vi "Client.vi"() -> ()   [LabVIEW 2020]
uses:
  Server/_support/Module/typedef/tcp-msg type.ctl
  <vilib>/event_ctls.llb/eventvkey.ctl
  a1c83761-5f2f-4742-9fa6-a9430ba65f56.vi
  <userlib>/_NEVSTOP/Communicable State Machine(CSM)/_Support/Common/Trim Single line Text.vi
  <userlib>/_NEVSTOP/Communicable State Machine(CSM)/AdvanceAPI/CSM - Keywords.vi
  <userlib>/_NEVSTOP/Communicable State Machine(CSM)/Communicable State Machine.lvlib
  <userlib>/_NEVSTOP/Communicable State Machine(CSM)/addons/API-String-Arugments-Support/API String Arguments Support.lvlib
  <userlib>/_NEVSTOP/Communicable State Machine(CSM)/addons/INI-Static-Variable-Support/INI-Static-Variable-Support.lvlib
  Server/_support/Module/CSM-TCP-Router.lvlib
panel:
  out "exit":bool
  out "Console":string
  in  "Command":string caption="$"
  out "To Who":string
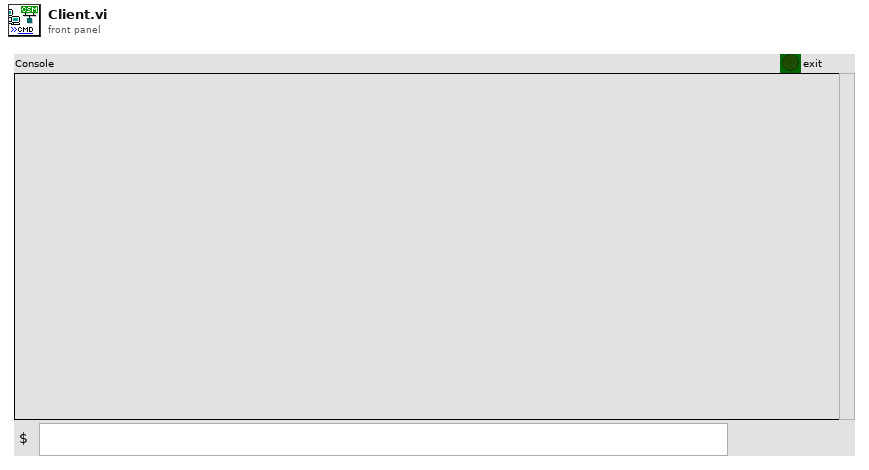
[diagram p1: front panel]
types:
  T1 = typedef "CSM-TCP-Router.lvlib/tcp-msg type.ctl" = enum8{"info", "error", "cmd", "resp", "async-resp", "status", "interrupt"}
  T2 = typedef "eventvkey.ctl" = enum16{"ASCII", "Enter", "Return", "Shift", "Ctrl", "Alt", "Cmd", "Opt", "Caps", "NumLock", "Clear", "Break", "Up", "Down", "Left", "Right", "Insert", "Delete", "Home", "End", "PageUp", "PageDown", "Escape", "Help", "Pause", "ScrollLock", "F1", "F2", "F3", "F4", "F5", "F6", "F7", "F8", "F9", "F10", "F11", "F12", "F13", "F14", "F15", "F16", "F17", "F18", "F19", "F20", "F21", "F22", "F23", "F24", "Play", "VolumeUp", "VolumeDown", "Mute", "Two Byte Char"}
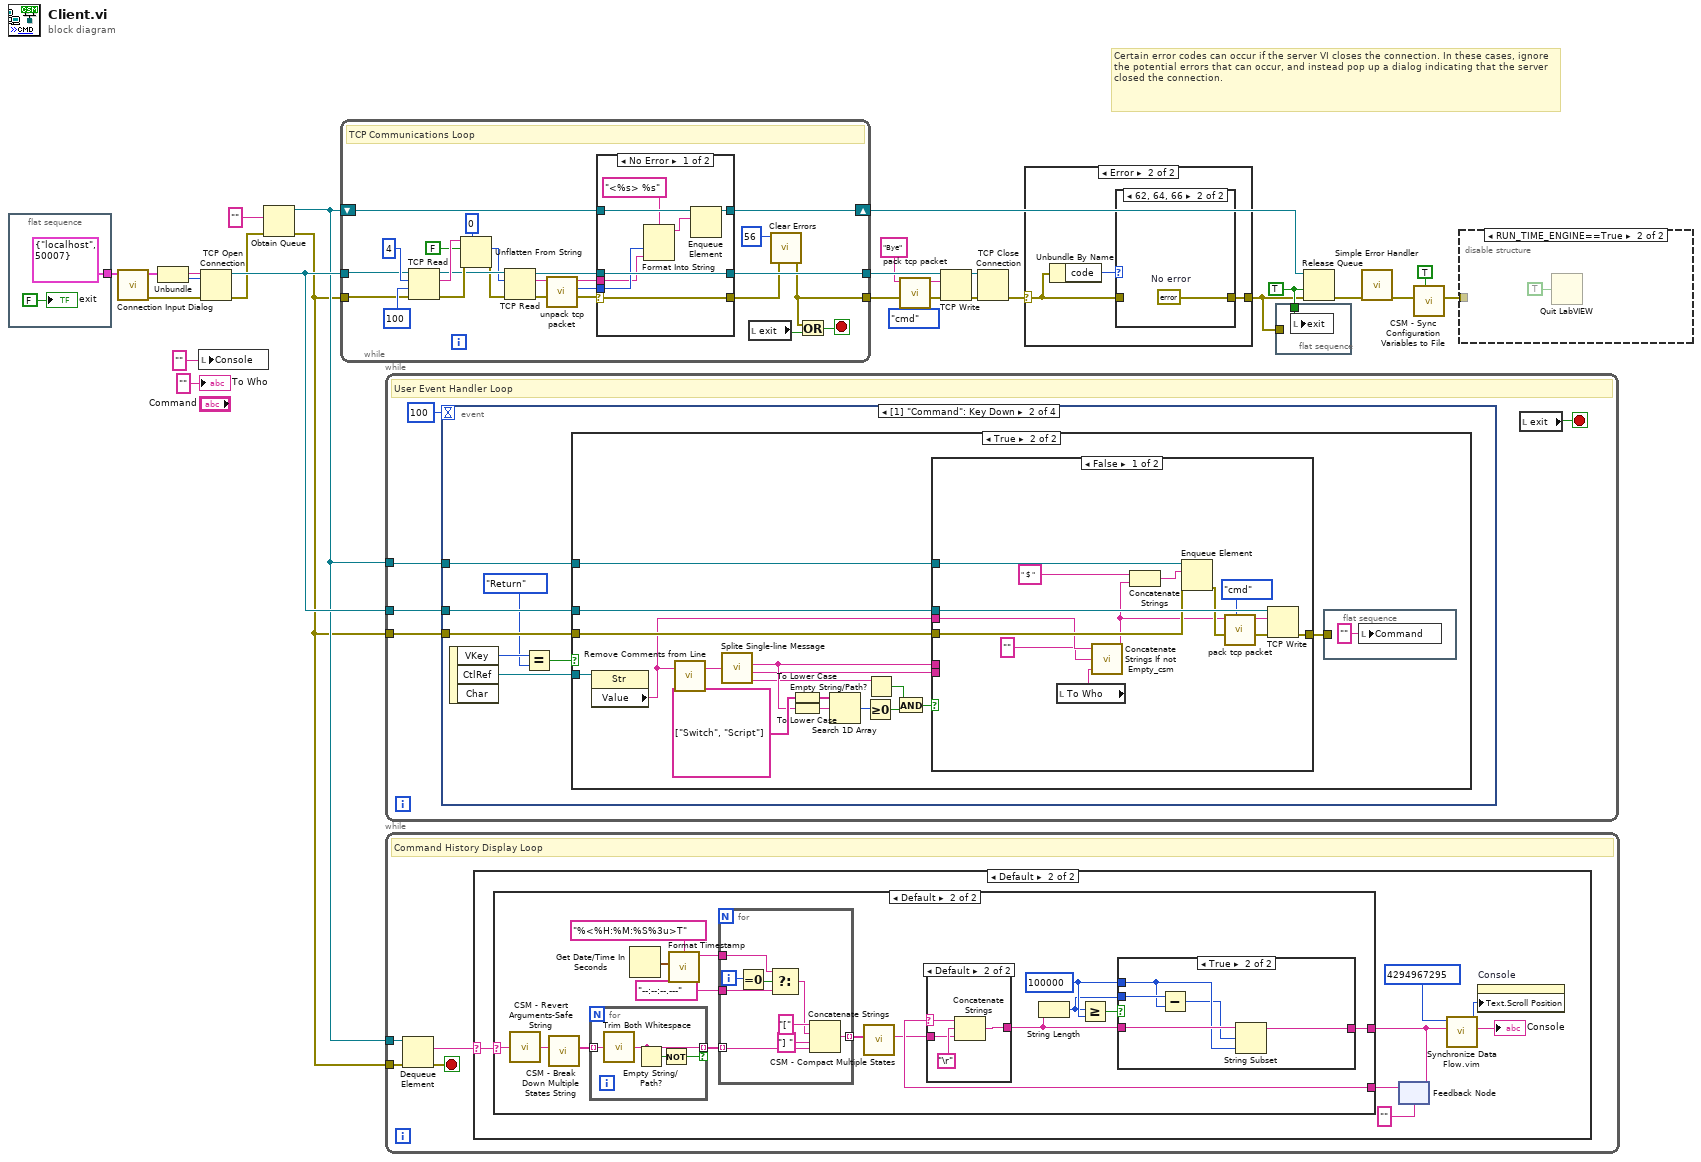
[diagram p0: block diagram]
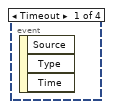
[diagram p7: hidden frame]
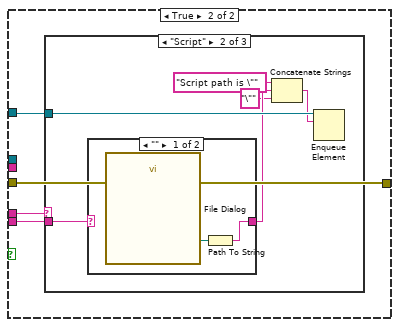
[diagram p9: hidden frame]
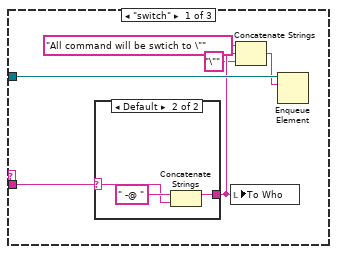
[diagram p10: hidden frame]
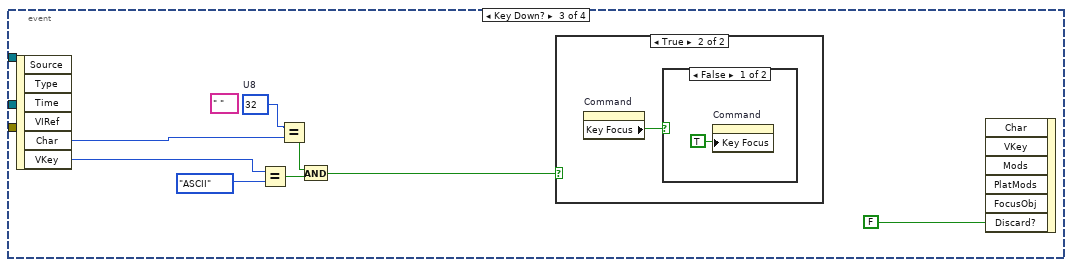
[diagram p14: hidden frame]
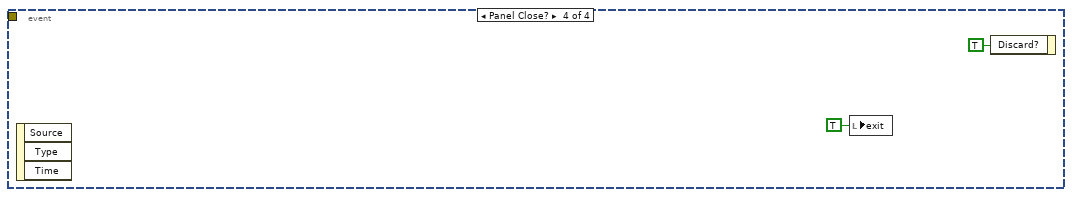
[diagram p17: hidden frame]
diagram:
  w6 = TRUE ("force destroy? (F)")
  # "Certain error codes can occur if the server VI closes the connection. In these cases, ignore the potential errors that can occur, and instead pop up a dialog indicating that the server closed the connection."
  n1 = flat-sequence {
    tunnel: [cluster{"IP Address":string, "Port":u16} {"IP Address"="localhost", "Port"=50007} ("Connection Info")] -> w16
    frame #0 {
      "exit" <- FALSE ("exit")
    }
  }
  n2 = call "Connection Input Dialog.vi"("Connection Info"=w16) -> ("Error out"=w15:errorcluster, "Connection Info output"=w14:cluster{"IP Address":string, "Port":u16})  [unwired: 9 in]
  n3 = Unbundle(w14) -> ("IP Address"=w13:string, "Port"=w12:u16)
  n4 = local write "Console"("" ("data out")) -> ()
  n5 = TCP Open Connection(address=w13, remote port or service name=w12, error in (no error)=w15) -> (connection ID=w21:refnum<k5>, error out=w9:errorcluster)  [unwired: 2 in]
  n6 = Obtain Queue(element data type="" ("name (unnamed)"), error in (no error)=w9) -> (queue out=w19:refnum<queue>, error out=w8:errorcluster)  [unwired: 3 in, 1 out]
  n7 = while {
    tunnel: w8 -> [w34]
    tunnel: w21 -> [w35]
    tunnel: [w53] -> w26
    tunnel: [w47] -> w24
    shift-right: [w49] -> w7
    shift-left: w19 -> [w50]
    stop <- w48 stop-if-true
    # "TCP Communications Loop"
    n8 = TCP Read(connection ID=w35, bytes to read=4, error in (no error)=w34, 9:100 ("timeout ms (1000)")) -> (connection ID out=w43:refnum<k5>, data out=w44:string, error out=w45:errorcluster)  [unwired: 1 in]
    n9 = Unflatten From String(type=0, binary string=w44, data includes array or string size? (T)=FALSE, error in (no error)=w45) -> (value=w41:i32, error out=w40:errorcluster)  [unwired: 2 out]
    n10 = TCP Read(connection ID=w43, bytes to read=w41, error in (no error)=w40) -> (connection ID out=w32:refnum<k5>, data out=w42:string, error out=w33:errorcluster)  [unwired: 2 in]
    n11 = call "unpack tcp packet.vi"("TCP Pack"=w42) -> ("tcp-message-type"=w30:T1, "String"=w31:string)  [unwired: 9 in]
    n12 = case shown="No Error" w33 {
      selector: w33 -> [w60 w64]
      tunnel: w32 -> [w61 w63]
      tunnel: [w61 w63] -> w53
      tunnel: [w60 w64] -> w52
      tunnel: w31 -> [w56 _]
      tunnel: w50 -> [w59 w62]
      tunnel: [w58 w62] -> w49
      tunnel: w30 -> [w57 _]
      frame No Error {
        n13 = Format Into String(format string="<%s> %s", w57, w56) -> (resulting string=w55:string)  [unwired: 2 in, 1 out]
        n14 = Enqueue Element(queue=w59, element=w55) -> (queue out=w58:refnum<queue>)  [unwired: 2 in, 2 out]
      }
      frame Error {
      }
    }
    n15 = local read "exit"() -> (w46:bool)
    n16 = call <vilib>:"Clear Errors.vi"("error in (no error)"=w52, "specific error code to clear (0: all)"=56) -> ("error out"=w47:errorcluster)  [unwired: 4 in, 1 out]
    n17 = Or(x=w47, y=w46) -> (x .or. y?=w48:bool)
  }
  n18 = while {
    tunnel: w21 -> [w69]
    tunnel: w8 -> [w68]
    tunnel: w19 -> [w66]
    stop <- w65 stop-if-true
    # "User Event Handler Loop"
    n19 = event shown="[1] \"Command\": Key Down" {
      selector: _ -> [_ _ _ _]
      dyn-events: _ -> [_ _ _ _]
      timeout: 100 -> [_ _ _ _]
      tunnel: w69 -> [_ w76 _ _]
      tunnel: w68 -> [_ w74 _ _]
      tunnel: w66 -> [_ w75 _ _]
      event Timeout {
        n20 = event-data() -> ()  [unwired: 1 in, 3 out]
      }
      event "Command": Key Down {
        n21 = event-data() -> ("VKey"=w72:T2, "CtlRef"=w73:refnum<vi>)  [unwired: 1 in, 1 out]
        n22 = Equal?(x=w72, y=eventvkey."Return") -> (x = y?=w70:bool)
        n23 = case shown="True" w70 {
          tunnel: w76 -> [_ w93]
          tunnel: w75 -> [_ w92]
          tunnel: w74 -> [_ w91]
          tunnel: w73 -> [_ w90]
          frame False {
          }
          frame True {
            n24 = property class="Str"(reference=w90) -> ("Value"=w87:string)  [unwired: 1 in, 2 out]
            n25 = call <userlib>:"Remove Comments from Line.vi"("single-line text"=w87) -> ("single-line text without comments"=w88:string)  [unwired: 2 in]
            n26 = call <userlib>:"Splite Single-line Message.vi"("single-line text"=w88) -> ("state"=w85:string, "args"=w77:string, "source/target"=w78:string)  [unwired: 6 in, 1 out]
            n27 = To Lower Case(string=string[] ["Switch", "Script"] ("hostname")) -> (all lower case string=w80:string[])
            n28 = To Lower Case(string=w85) -> (all lower case string=w79:string)
            n29 = Search 1D Array(1D array=w80, element=w79) -> (index of element=w84:i32)  [unwired: 1 in]
            n30 = Greater Or Equal To 0?(x=w84) -> (x >= 0?=w83:bool)
            n31 = Empty String/Path?(string/path=w78) -> (empty?=w82:bool)
            n32 = And(x=w82, y=w83) -> (x .and. y?=w81:bool)
            n33 = case shown="False" w81 {
              tunnel: w93 -> [w106 _]
              tunnel: w92 -> [w105 w109]
              tunnel: w91 -> [w101 w110]
              tunnel: [w100 w110] -> w89
              tunnel: w87 -> [w99 _]
              tunnel: w85 -> [_ w107]
              tunnel: w77 -> [_ w108]
              frame False {
                n34 = local read "To Who"() -> (w96:string)
                n35 = call <userlib>:"Concatenate Strings If not Empty_csm.vi"("String"=w96, "seperator(:)"="", "prefix"=w99) -> ("result"=w98:string)  [unwired: 2 in]
                n36 = Concatenate Strings(" $ " ("string"), w98) -> (w103:string)
                n37 = Enqueue Element(queue=w105, element=w103, error in (no error)=w101) -> (error out=w102:errorcluster)  [unwired: 1 in, 2 out]
                n38 = call "pack tcp packet.vi"("tcp-message-type"=tcp-msg_type."cmd", "String"=w98) -> ("TCP Pack"=w95:string)  [unwired: 9 in]
                n39 = TCP Write(connection ID=w106, data in=w95, error in (no error)=w102) -> (error out=w100:errorcluster)  [unwired: 1 in, 2 out]
              }
              frame True {
                n40 = case shown="\"Script\"" w107 {
                  tunnel: w109 -> [w115 w124 _]
                  tunnel: w108 -> [w116 w125 _]
                  frame "switch" {
                    n41 = case shown="Default" w116 {
                      selector: w116 -> [_ w117]
                      tunnel: [_ w118] -> w114
                      frame "" {
                      }
                      frame Default {
                        n42 = Concatenate Strings(" -@ " ("To Who"), w117) -> (w118:string)
                      }
                    }
                    n43 = local write "To Who"(w114) -> ()
                    n44 = Concatenate Strings("All command will be swtich to \"" ("string"), w114, "\"" ("string")) -> (w113:string)
                    n45 = Enqueue Element(queue=w115, element=w113) -> ()  [unwired: 2 in, 3 out]
                  }
                  frame "Script" {
                    n46 = case shown="\"\"" w125 {
                      selector: w125 -> [_ w128]
                      tunnel: [w126 w128] -> w123
                      frame "" {
                        n47 = call "File Dialog"() -> ("selected path"=w127:path)  [unwired: 12 in, 3 out]
                        n48 = Path To String(path=w127) -> (string=w126:string)
                      }
                      frame Default {
                      }
                    }
                    n49 = Concatenate Strings("Script path is \"" ("string"), w123, "\"" ("string")) -> (w122:string)
                    n50 = Enqueue Element(queue=w124, element=w122) -> ()  [unwired: 2 in, 3 out]
                  }
                  frame Default {
                  }
                }
              }
            }
            n51 = flat-sequence {
              tunnel: w89 -> [_]
              frame #0 {
                n52 = local write "Command"("" ("Command")) -> ()
              }
            }
          }
        }
      }
      event Key Down? {
        (unwired) " "
        w132 = u8 32  # U8
        n53 = event-data() -> ("Char"=w133:i16, "VKey"=w135:T2)  [unwired: 1 in, 4 out]
        n54 = Equal?(x=w135, y=eventvkey."ASCII" ("VKey")) -> (x = y?=w134:bool)
        n55 = Equal?(x=w132, y=w133) -> (x = y?=w131:bool)
        n56 = And(x=w131, y=w134) -> (x .and. y?=w130:bool)
        n57 = case shown="True" w130 {
          frame False {
          }
          frame True {
            n58 = property on="Command" class="Str"() -> ("Key Focus"=w138:bool)  [unwired: 2 in, 2 out]
            n59 = case shown="False" w138 {
              frame False {
                n60 = property on="Command" class="Str"("Key Focus"=TRUE) -> ()  [unwired: 2 in, 2 out]
              }
              frame True {
              }
            }
          }
        }
        n61 = event-data("Discard?"=FALSE) -> ()  [unwired: 6 in, 1 out]
      }
      event Panel Close? {
        n62 = event-data() -> ()  [unwired: 1 in, 3 out]
        n63 = local write "exit"(TRUE ("exit")) -> ()
        n64 = event-data("Discard?"=TRUE) -> ()  [unwired: 1 in, 1 out]
      }
    }
    n65 = local read "exit"() -> (w65:bool)
  }
  n66 = while {
    tunnel: w8 -> [w144]
    tunnel: w19 -> [w145]
    stop <- w143 stop-if-true
    # "Command History Display Loop"
    n67 = Dequeue Element(queue=w145, error in (no error)=w144) -> (element=w142:string, error out=w143:errorcluster)  [unwired: 1 in, 2 out]
    n68 = case shown="Default" w142 {
      selector: w142 -> [_ w149]
      frame "" {
      }
      frame Default {
        n69 = feedback #1("") -> (w152:string)
        n70 = case shown="Default" w149 {
          selector: w149 -> [_ w158]
          tunnel: w152 -> [w153 w168]
          tunnel: [w153 w169] -> w150
          frame "" {
          }
          frame Default {
            w166 = 100000 ("length")
            n71 = call <userlib>:"CSM - Revert Arguments-Safe String.vi"("Safe Argurment String"=w158) -> ("Origin Argurment String"=w160:string)  [unwired: 8 in]
            n72 = call <userlib>:"CSM - Break Down Multiple States String.vi"("States"=w160) -> ("Multiple States"=w159:string[])  [unwired: 10 in]
            n73 = for {
              tunnel: w159 -> [w182] mode=indexing
              tunnel: [w181] -> w157 mode=indexing if=w179
              n74 = call <userlib>:"Trim Both Whitespace.vi"("string"=w182) -> ("trimmed string"=w181:string)  [unwired: 1 in]
              n75 = Empty String/Path?(string/path=w181) -> (empty?=w180:bool)
              n76 = Not(x=w180) -> (.not. x?=w179:bool)
            }
            n77 = Get Date/Time In Seconds() -> (seconds since 1Jan1904=w161:timestamp)
            n78 = call <userlib>:"Format Timestamp.vi"("timestamp"=w161, "format string"="%<%H:%M:%S%3u>T") -> ("String"=w163:string)  [unwired: 9 in]
            n79 = for {
              tunnel: w163 -> [w172]
              tunnel: [w176] -> w156 mode=indexing
              tunnel: w157 -> [w175] mode=indexing
              tunnel: "--:--:--.---" ("format string") -> [w171]
              i -> [w174]
              n80 = Equal To 0?(x=w174) -> (x = 0?=w173:bool)
              n81 = Select(t=w172, s=w173, f=w171) -> (s? t:f=w170:string)
              n82 = Concatenate Strings("[" ("string"), w170, "] " ("string"), w175) -> (w176:string)
            }
            n83 = call <userlib>:"CSM - Compact Multiple States.vi"("Multiple States"=w156) -> ("States"=w155:string)  [unwired: 9 in]
            n84 = case shown="Default" w168 {
              selector: w168 -> [_ w191]
              tunnel: [w189 w192] -> w167
              tunnel: w155 -> [w189 w190]
              frame "" {
              }
              frame Default {
                n85 = Concatenate Strings(w191, "\r", w190) -> (w192:string)
              }
            }
            n86 = String Length(string=w167) -> (length=w164:i32)
            n87 = Greater Or Equal?(x=w164, y=w166) -> (x >= y?=w165:bool)
            n88 = case shown="True" w165 {
              tunnel: [w183 w188] -> w169
              tunnel: w167 -> [w183 w187]
              tunnel: w166 -> [_ w185]
              tunnel: w164 -> [_ w186]
              frame False {
              }
              frame True {
                n89 = Subtract(x=w186, y=w185) -> (x-y=w184:i32)
                n90 = String Subset(string=w187, offset (0)=w184, length (rest)=w185) -> (substring=w188:string)
              }
            }
          }
        }
        n91 = feedback-in #1(w150) -> ()
        n92 = call "Synchronize Data Flow.vim"("input 2"=w150, "input 1"=u32 4294967295 ("Text.Scroll Position")) -> ("output 2"=→"Console":string, "output 1"=w146:u32)  [unwired: 2 in, 2 out]
        n93 = property on="Console" class="Str"("Text.Scroll Position"=w146) -> ()  [unwired: 2 in, 2 out]
      }
    }
  }
  n94 = call "pack tcp packet.vi"("tcp-message-type"=tcp-msg_type."cmd", "String"="Bye") -> ("TCP Pack"=w2:string)  [unwired: 9 in]
  n95 = TCP Write(connection ID=w26, data in=w2, error in (no error)=w24) -> (connection ID out=w27:refnum<k5>, error out=w25:errorcluster)  [unwired: 1 in, 1 out]
  n96 = TCP Close Connection(connection ID=w27, error in (no error)=w25) -> (error out=w5:errorcluster)  [unwired: 1 in, 1 out]
  n97 = case shown="Error" w5 {
    selector: w5 -> [w194 w196]
    tunnel: [w194 w195] -> w3
    frame No Error {
    }
    frame Error {
      n98 = Unbundle By Name(w196) -> ("code"=w197:i32)
      n99 = case shown="62, 64, 66" w197 {
        tunnel: w196 -> [w198 _]
        tunnel: [w198 w199] -> w195
        frame Default {
        }
        frame 62, 64, 66 {
          w199 = errorcluster {"status"=FALSE, "code"=0, "source"=""}  # No error
        }
      }
    }
  }
  n100 = flat-sequence {
    tunnel: w6 -> [w200]
    tunnel: w3 -> [_]
    frame #0 {
      n101 = local write "exit"(w200) -> ()
    }
  }
  n102 = Release Queue(queue=w7, force destroy? (F)=w6, error in (no error)=w3) -> (error out=w4:errorcluster)  [unwired: 2 out]
  n103 = call <vilib>:"Simple Error Handler.vi"("error in (no error)"=w4) -> ("error out"=w17:errorcluster)  [unwired: 4 in, 4 out]
  n104 = call <userlib>:"CSM - Sync Configuration Variables to File.vi"("All Temp Variable to Default Ini(F)"=TRUE, "error in (no error)"=w17) -> ("error out"=w11:errorcluster)  [unwired: 7 in]
  n105 = disable-structure shown="RUN_TIME_ENGINE==True" {
    disable-tunnel: w11 -> [_ _]
    frame condition #0 (active) {
    }
    frame condition #1 {
      n106 = Quit LabVIEW(quit? (T)=TRUE) -> ()
    }
  }
  "To Who" <- "" ("hostname")
